vi "Read Async Raw Data.vi"(5 "Component ID":u8, 7 "FPGA Interface":refnum<class "FPGA Interface.lvclass">, 8 "error in (no error)":errorcluster, 10 "Async Message":refnum<class "Async Message.lvclass">, 11 "Bus Controller in":refnum<class "Bus Controller.lvclass">) -> (0 "error out":errorcluster, 1 "Parameter Data":u64[](array[numeric]), 2 "Parameters":string[](array[string]), 3 "Bus Controller out":refnum<class "Bus Controller.lvclass">)   [LabVIEW 2020, in "BCI-1553 API.lvlib" / "Bus Controller.lvclass"]
doc: "Reads raw parameter data associated with the argument Asynchronous Message. An Asynchronous Message must be sent before this method will return valid data."
uses:
  Bus Controller.lvclass
  Dependencies/FPGA Interface/FPGA Interface.lvclass
  Frames & Messages/Async Message/Async Message.lvclass
  Bus Controller.lvclass/Bus Controller.ctl
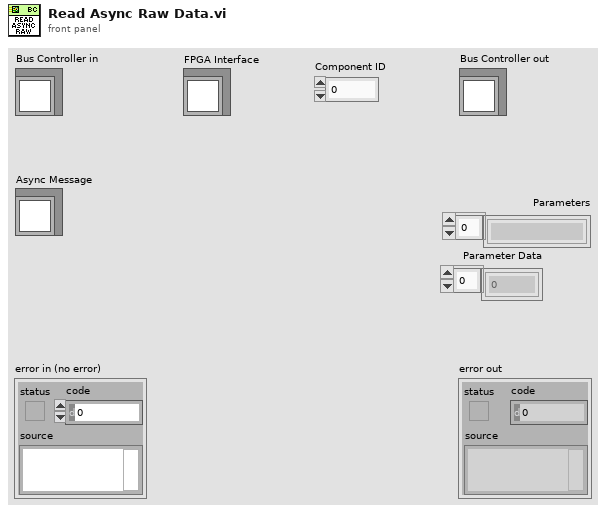
[diagram p1: front panel]
types:
  T1 = typedef "BCI-1553 API.lvlib/Async Message Pointers.ctl" = cluster{"HP Async Control Addresses":u16[], "HP Async Data Addresses":u16[], "LP Async Control Addresses":u16[], "LP Async Data Addresses":u16[]}
  T2 = typedef "BCI-1553 API.lvlib/Async Payload.ctl" = cluster{"Configuration Address":u16, "Configuration":u16[], "Data Address":u16, "Data":u16[], "Trigger Command":u16, "Command Type":enum16{"Transmit", "Receive"}}
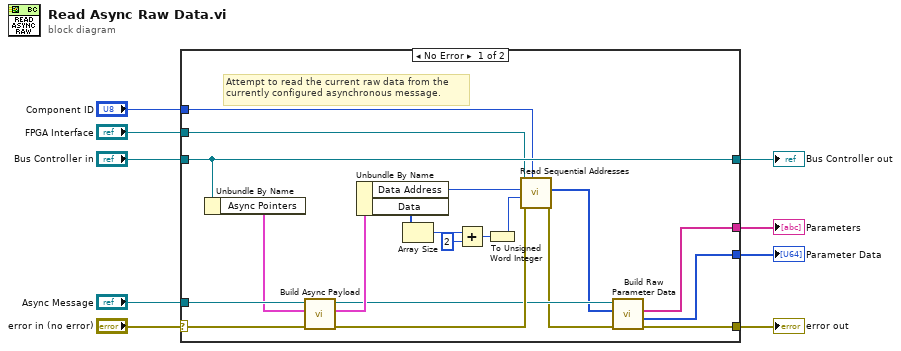
[diagram p0: block diagram]
diagram:
  n1 = case shown="No Error" "error in (no error)" {
    selector: "error in (no error)" -> [w27 w31]
    tunnel: [w12 w31] -> w3
    tunnel: [w26 w30] -> w4
    tunnel: "Bus Controller in" -> [w26 w30]
    tunnel: "Async Message" -> [w29 _]
    tunnel: "FPGA Interface" -> [w24 _]
    tunnel: "Component ID" -> [w23 _]
    tunnel: [w11 _] -> w2
    tunnel: [w10 _] -> w1
    frame No Error {
      # "Attempt to read the current raw data from the\ncurrently configured asynchronous message."
      n2 = Unbundle By Name(w26) -> ("Async Pointers"=w28:T1)
      n3 = call-dynamic "Build Async Payload.vi"("error in (no error)"=w27, "Async Pointers"=w28, "Async Message in"=w29) -> ("error out"=w21:errorcluster, "Async Payload"=w25:T2, "Async Message out"=w15:refnum<class "Async Message.lvclass">)  [unwired: 6 in]
      n4 = Unbundle By Name(w25) -> ("Data Address"=w22:u16, "Data"=w20:u16[])
      n5 = Array Size(array=w20) -> (size(s)=w19:i32)
      n6 = Add(x=w19, y=2) -> (x+y=w17:i32)
      n7 = To Unsigned Word Integer(number=w17) -> (unsigned 16bit integer=w16:u16)
      n8 = call-dynamic "Read Sequential Addresses.vi"("Target IC (1-8)"=w23, "error in (no error)"=w21, "Addresses to Read"=w16, "Starting Address"=w22, "FPGA Interface in"=w24) -> ("error out"=w13:errorcluster, "Data"=w14:u16[])  [unwired: 5 in]
      n9 = call-dynamic "Build Raw Parameter Data.vi"("error in (no error)"=w13, "FPGA Data"=w14, "Async Message in"=w15) -> ("error out"=w12:errorcluster, "Parameter Data"=w10:u64[], "Parameters"=w11:string[])  [unwired: 5 in, 1 out]
    }
    frame Error {
    }
  }
  "error out" <- w3
  "Bus Controller out" <- w4
  "Parameters" <- w2
  "Parameter Data" <- w1
